vi "Utilities.Buffer.String.vi"(8 "error in (no error)":errorcluster, 10 "buffer in":string, 11 "minimum size":i64) -> (0 "error out":errorcluster, 2 "buffer out":string)   [LabVIEW 2016, in "VeriStand Data.lvlib"]
uses:
  VeriStand Data.lvlib
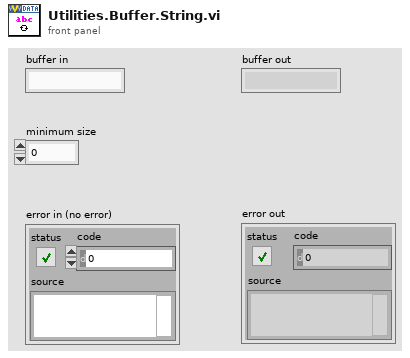
[diagram p1: front panel]
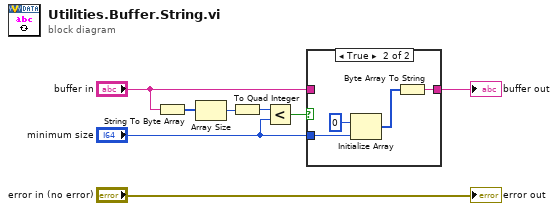
[diagram p0: block diagram]
diagram:
  n1 = String To Byte Array(string="buffer in") -> (unsigned byte array=w3:u8[])
  n2 = Array Size(array=w3) -> (size(s)=w2:i32)
  n3 = To Quad Integer(1:w2) -> (0:w4:i64)
  n4 = Less?(x=w4, y="minimum size") -> (x < y?=w7:bool)
  n5 = case shown="True" w7 {
    tunnel: "buffer in" -> [w9 _]
    tunnel: "minimum size" -> [_ w12]
    tunnel: [w9 w10] -> w6
    frame False {
    }
    frame True {
      n6 = Initialize Array(u8 0 ("element"), w12) -> (w11:u8[])
      n7 = Byte Array To String(unsigned byte array=w11) -> (string=w10:string)
    }
  }
  "buffer out" <- w6
  "error out" <- "error in (no error)"
